vi "Fick to RV in 1 plane.vi"(4 "Fick IN":dbl[][](array[numeric])) -> (1 "Angle OUT":dbl[][](array[numeric]))   [LabVIEW 2013]
panel:
  # "This formula can only be used if \nthe rotation is purely in one plane"
  # "alpha_RV = 2* atan(alpha_F)"
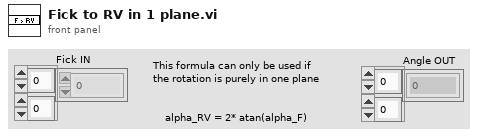
[diagram p1: front panel]
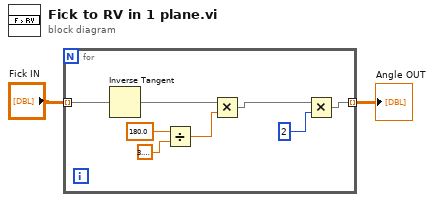
[diagram p0: block diagram]
diagram:
  n1 = for {
    tunnel: [w8] -> w1 mode=indexing
    tunnel: "Fick IN" -> [w10] mode=indexing
    n2 = Inverse Tangent(1:w10) -> (0:w7:dbl[])
    n3 = Divide(x=180.0, y=3.141592653589793) -> (x/y=w4:dbl)
    n4 = Multiply(x=w7, y=w4) -> (x*y=w3:dbl[])
    n5 = Multiply(x=w3, y=2) -> (x*y=w8:dbl[])
  }
  "Angle OUT" <- w1
